vi "ScanMoveDone.vi"(8 "error in (no error)":errorcluster, 11 "Spectroscopy_Controller in":refnum<class "Spectroscopy_Controller.lvclass">) -> (0 "error out":errorcluster, 3 "Spectroscopy_Controller out":refnum<class "Spectroscopy_Controller.lvclass">)   [LabVIEW 2023, in "Spectroscopy_Controller.lvlib" / "Spectroscopy_Controller.lvclass"]
uses:
  Spectroscopy_Controller.lvclass
  Spectroscopy_Controller.lvclass/Spectroscopy_Controller.ctl
  <vilib>/ActorFramework/Message Enqueuer/Message Enqueuer.lvclass/Message Enqueuer.ctl
  <vilib>/ActorFramework/Message Enqueuer/Enqueue.vi
  UIs/Camera_Controller/Camera_Controller Messages/External_Acq Msg/External_Acq Msg.lvclass
  <vilib>/ActorFramework/Message Priority Queue/Priority Enqueue.vi
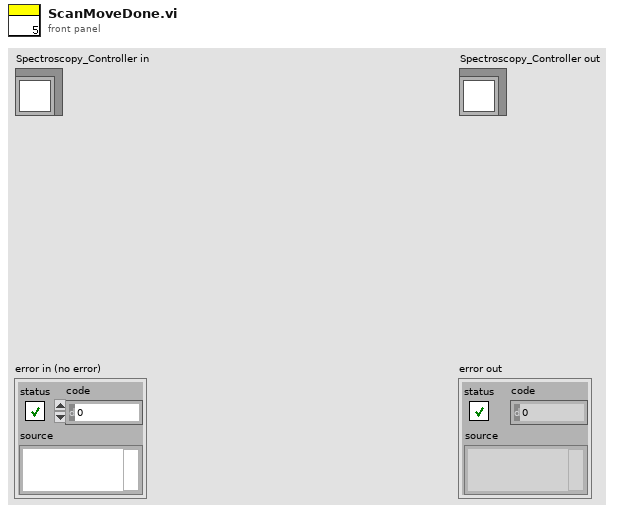
[diagram p1: front panel]
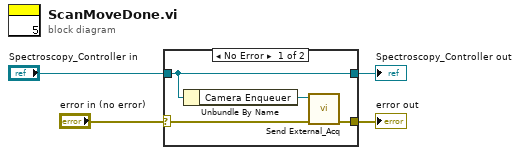
[diagram p0: block diagram]
diagram:
  n1 = case shown="No Error" "error in (no error)" {
    selector: "error in (no error)" -> [w6 w10]
    tunnel: [w5 w10] -> w3
    tunnel: [w7 w9] -> w1
    tunnel: "Spectroscopy_Controller in" -> [w7 w9]
    frame No Error {
      n2 = Unbundle By Name(w7) -> ("Camera Enqueuer"=w8:refnum<class "Message Enqueuer.lvclass">)
      n3 = call "Send External_Acq.vi"("error in (no error)"=w6, "Message Enqueuer"=w8) -> ("error out"=w5:errorcluster)  [unwired: 8 in, 1 out]
    }
    frame Error {
    }
  }
  "error out" <- w3
  "Spectroscopy_Controller out" <- w1
